vi "DRAM Pack data.vi"(9 "Data input":u32, 10 "Adress input":u32, 11 "Input valid?":bool=TRUE) -> (0 "Array":u32[](array[numeric]), 3 "Address output":u32, 4 "output":bool=TRUE)   [LabVIEW 2015]
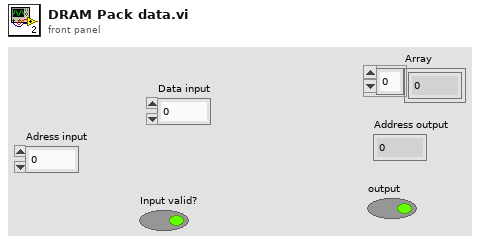
[diagram p1: front panel]
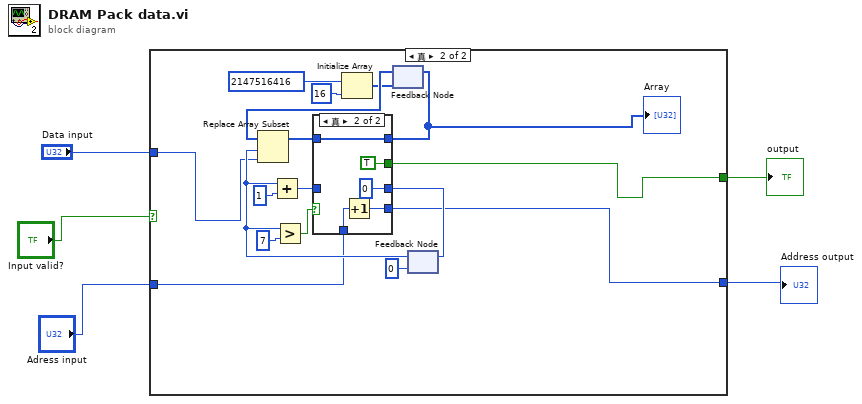
[diagram p0: block diagram]
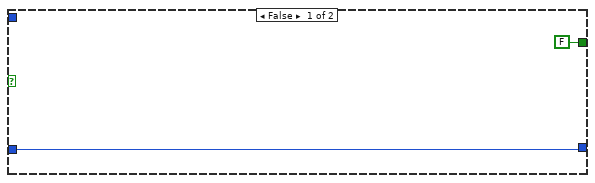
[diagram p2: hidden frame]
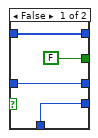
[diagram p3: hidden frame]
diagram:
  n1 = case shown="真" "Input valid?" {
    tunnel: [FALSE w11] -> w4
    tunnel: "Adress input" -> [w6 w10]
    tunnel: "Data input" -> [_ w9]
    tunnel: [w6 w8] -> w1
    frame False {
    }
    frame True {
      n2 = Initialize Array(u32 2147516416 ("element"), 16 ("dimension size")) -> (w15:u32[])
      n3 = feedback #1(w15) -> (w23:u32[])
      n4 = feedback #2(u32 0) -> (w22:u32)
      n5 = Replace Array Subset(array=w23, new element=w9, index=w22) -> (w19:u32[])
      n6 = Add(x=w22, y=u32 1) -> (x+y=w20:u32)
      n7 = Greater?(x=w22, y=u32 7) -> (0:w18:bool)
      n8 = case shown="真" w18 {
        tunnel: w20 -> [w28 _]
        tunnel: [w28 u32 0] -> w14
        tunnel: w19 -> [w27 w32]
        tunnel: [w27 w32] -> w12
        tunnel: w10 -> [w26 w31]
        tunnel: [w26 w30] -> w8
        tunnel: [FALSE TRUE] -> w11
        frame False {
        }
        frame True {
          n9 = Increment(x=w31) -> (x+1=w30:u32)
        }
      }
      "Array" <- w12
      n10 = feedback-in #1(w12) -> ()
      n11 = feedback-in #2(w14) -> ()
    }
  }
  "output" <- w4
  "Address output" <- w1
